vi "innit_message_queue.vi"   [LabVIEW 2023]
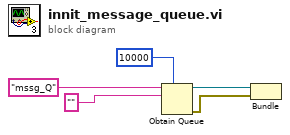
[diagram p0: block diagram]
diagram:
  n1 = Obtain Queue(max queue size (-1, unlimited)=10000, name (unnamed)="mssg_Q", element data type="") -> (queue out=w2:refnum<queue>, error out=w1:errorcluster)  [unwired: 2 in, 1 out]
  n2 = Bundle("queue out"=w2, "error out"=w1) -> ()  [unwired: 1 in, 1 out]
